vi "Test.vi"() -> ()   [LabVIEW 2024, in "Ni-Scope Digitizer.lvclass"]
uses:
  Ni-Scope Digitizer.lvclass
  Ni-Scope Digitizer.lvclass/Ni-Scope Digitizer.ctl
  Instruments/Pulse Driver/Pusle Driver Configuration.ctl
panel:
  out "Fetch Relative To":i32=477
  out "Samples per channel":i32
  out "Pretrigger samples":i32
  out "t0":dbl format="%#_6e"
  out "dt":dbl format="%#_6e"
  in  "Pulse Configuration":T1={"Post-trigger delay"=-0.01, "Post-trigger duration"=0.1, "Rate"=1000000.0, "Ranges"=[10.0], "Re-name channels"=[], "Active channels"="0:1", "External clock"=FALSE} {"Rate" format="%#_8pHz"; "Post-trigger duration" format="%#_6ps"; "Post-trigger delay" format="%#_6ps"; "Ranges" format="%#_6pV"}
  in  "Device name":refnum<k15>="5105-PCI"
  in  "Ni-Scope Digitizer in":refnum<class "Ni-Scope Digitizer.lvclass">
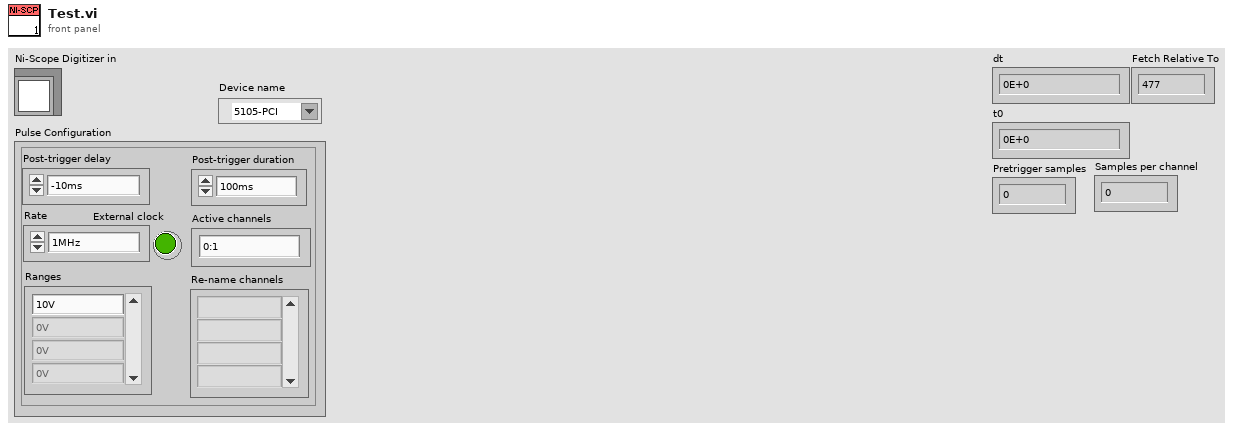
[diagram p1: front panel]
types:
  T1 = typedef "Pusle Driver Configuration.ctl" = cluster{"Post-trigger delay":dbl, "Post-trigger duration":dbl, "Rate":dbl, "Ranges":dbl[], "Re-name channels":string[], "Active channels":string, "External clock":bool}
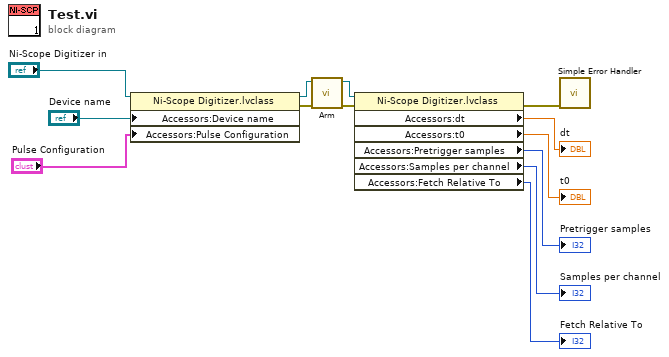
[diagram p0: block diagram]
diagram:
  n1 = property class="Ni-Scope Digitizer.lvclass"(reference="Ni-Scope Digitizer in", "Accessors:Device name"="Device name", "Accessors:Pulse Configuration"="Pulse Configuration") -> (reference out=w11:refnum<class "Ni-Scope Digitizer.lvclass">, error out=w10:errorcluster)  [unwired: 1 in]
  n2 = call-dynamic "Arm.vi"("error in (no error)"=w10, "Pulse Driver in"=w11) -> ("error out"=w7:errorcluster, "Pulse Driver out"=w8:refnum<class "Ni-Scope Digitizer.lvclass">)  [unwired: 7 in, 1 out]
  n3 = property class="Ni-Scope Digitizer.lvclass"(reference=w8, error in=w7) -> (error out=w1:errorcluster, "Accessors:dt"=→"dt":dbl, "Accessors:t0"=→"t0":dbl, "Accessors:Pretrigger samples"=→"Pretrigger samples":i32, "Accessors:Samples per channel"=→"Samples per channel":i32, "Accessors:Fetch Relative To"=→"Fetch Relative To":i32)  [unwired: 1 out]
  n4 = call <vilib>:"Simple Error Handler.vi"("error in (no error)"=w1) -> ()  [unwired: 4 in, 5 out]
